vi "Shooter Profile.vi"(10 "Target V (RPM)":dbl, 11 "Max Accel (RPM)":dbl=50.0) -> (3 "vel_for_shooterFF (RPM)":dbl)   [LabVIEW 2015]
panel:
  out "Shooter Velocity Chart":dbl(graph)
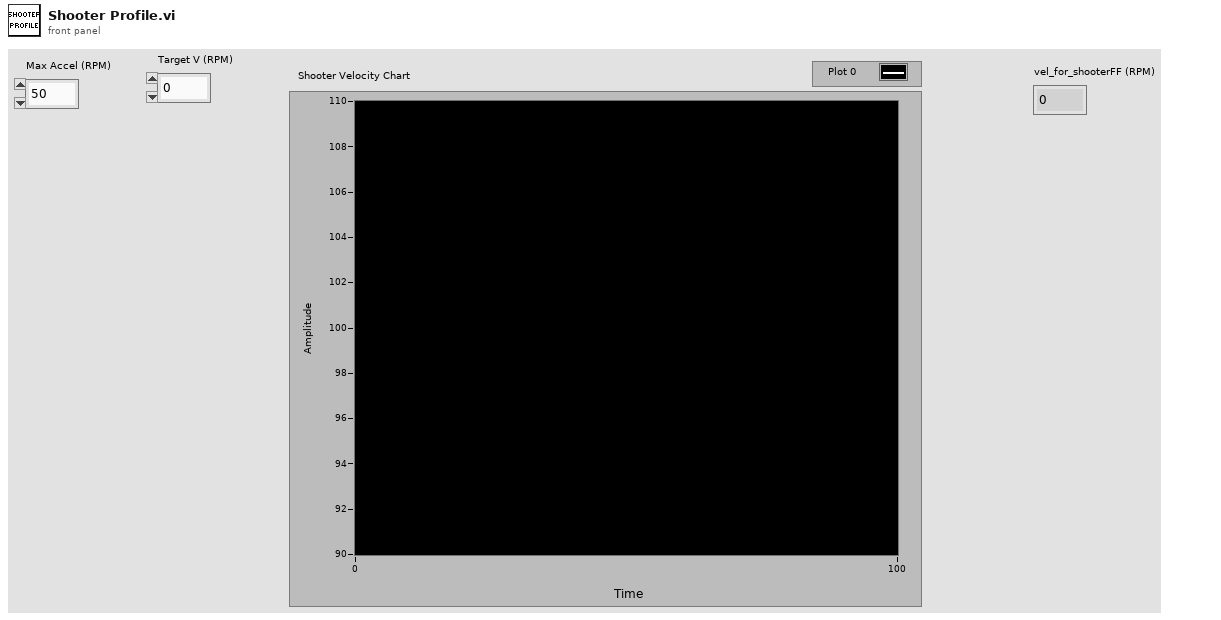
[diagram p1: front panel]
types:
  T1 = enum16{"v_accel", "v_naccel", "v_cruise", "v_rest"}
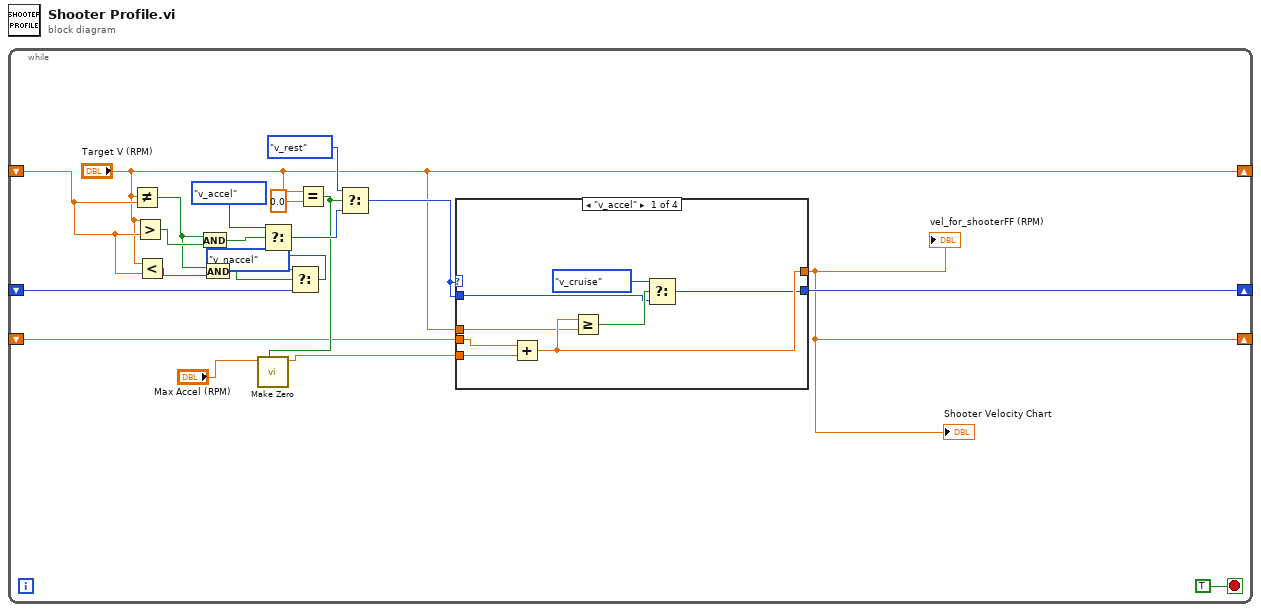
[diagram p0: block diagram]
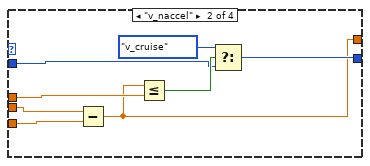
[diagram p2: hidden frame]
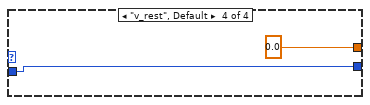
[diagram p4: hidden frame]
diagram:
  n1 = while {
    shift-right: ["Target V (RPM)"] -> _
    shift-left: _ -> [w17]
    shift-right: [w1] -> _
    shift-left: _ -> [w7]
    shift-right: [w4] -> _
    shift-left: _ -> [w3]
    stop <- TRUE stop-if-true
    n2 = Not Equal?(x="Target V (RPM)", y=w17) -> (x != y?=w18:bool)
    n3 = Greater?(x="Target V (RPM)", y=w17) -> (0:w21:bool)
    n4 = Less?(x="Target V (RPM)", y=w17) -> (x < y?=w16:bool)
    n5 = And(x=w18, y=w21) -> (x .and. y?=w20:bool)
    n6 = And(x=w18, y=w16) -> (x .and. y?=w15:bool)
    n7 = Select(t=T1."v_naccel", s=w15, f=w3) -> (s? t:f=w10:T1)
    n8 = Select(t=T1."v_accel", s=w20, f=w10) -> (s? t:f=w11:T1)
    n9 = Equal?(x="Target V (RPM)", y=0.0) -> (x = y?=w8:bool)
    n10 = call "Make Zero.vi"("Boolean"=w8, "Input"="Max Accel (RPM)") -> ("Output"=w6:dbl)  [unwired: 7 in]
    n11 = Select(t=T1."v_rest", s=w8, f=w11) -> (s? t:f=w5:T1)
    n12 = case shown="\"v_accel\"" w5 {
      tunnel: [w28 w31 w40 0.0] -> w1
      tunnel: w7 -> [w30 w33 w40 _]
      tunnel: w6 -> [w29 w32 _ _]
      tunnel: "Target V (RPM)" -> [w27 w34 _ _]
      tunnel: w5 -> [w25 w36 w39 w41]
      tunnel: [w24 w35 w39 w41] -> w4
      frame "v_accel" {
        n13 = Add(x=w30, y=w29) -> (x+y=w28:dbl)
        n14 = Greater Or Equal?(x=w28, y=w27) -> (x >= y?=w26:bool)
        n15 = Select(t=T1."v_cruise", s=w26, f=w25) -> (s? t:f=w24:T1)
      }
      frame "v_naccel" {
        n16 = Subtract(x=w33, y=w32) -> (x-y=w31:dbl)
        n17 = Less Or Equal?(x=w31, y=w34) -> (x <= y?=w38:bool)
        n18 = Select(t=T1."v_cruise", s=w38, f=w36) -> (s? t:f=w35:T1)
      }
      frame "v_cruise" {
      }
      frame "v_rest", Default {
      }
    }
    "vel_for_shooterFF (RPM)" <- w1
    "Shooter Velocity Chart" <- w1
  }
